vi "Set JSON Config.vi"(8 "error in (no error)":errorcluster, 10 "<JSON>Config>":string, 11 "CFG Base in":refnum<class "CFG JSON Base.lvclass">) -> (0 "error out":errorcluster, 3 "CFG Base out":refnum<class "CFG JSON Base.lvclass">)   [LabVIEW 2023, in "HAL GOOP4.lvlib" / "CFG JSON Base.lvclass"]
uses:
  CFG JSON Base.lvclass
  CFG JSON Base.lvclass/CFG JSON Base.ctl
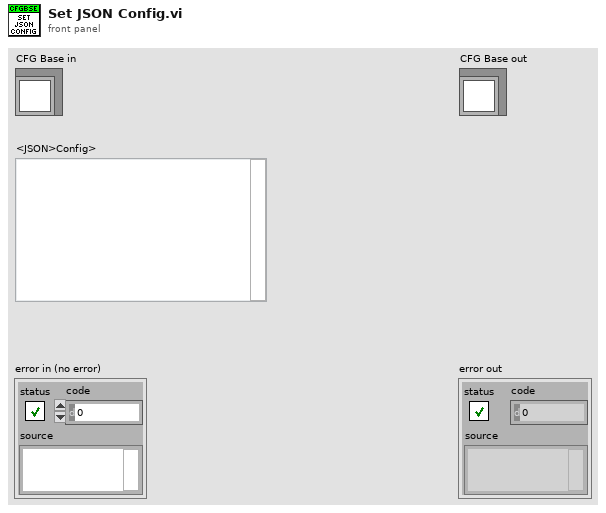
[diagram p1: front panel]
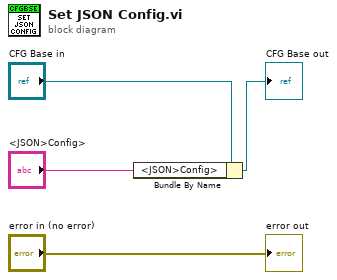
[diagram p0: block diagram]
diagram:
  n1 = Bundle By Name(cluster="CFG Base in", "<JSON>Config>"="<JSON>Config>") -> (→"CFG Base out":refnum<class "CFG JSON Base.lvclass">)
  "error out" <- "error in (no error)"
